vi "FPGA_EncoderOpen & Configure.vi"(4 "IndexActiveHigh":bool=TRUE, 5 "IndexSource":T1={"DevStatus"={"status"=FALSE, "code"=0, "source"=""}, "AnalogTriggerMode?"=FALSE, "DigitalMode"={"DIO Channel"=enum."Disabled"}, "AnalogTriggerMode"={"AnalogTriggerIndex"=enum."Trig 0", "OutputType"=enum."InWindow"}}, 6 "Reverse?":bool, 7 "IndexEdgeSensitive":bool, 8 "error in":errorcluster, 9 "BSource":T1={"DevStatus"={"status"=FALSE, "code"=0, "source"=""}, "AnalogTriggerMode?"=FALSE, "DigitalMode"={"DIO Channel"=enum."Disabled"}, "AnalogTriggerMode"={"AnalogTriggerIndex"=enum."Trig 0", "OutputType"=enum."InWindow"}}, 10 "ASource":T1={"DevStatus"={"status"=FALSE, "code"=0, "source"=""}, "AnalogTriggerMode?"=FALSE, "DigitalMode"={"DIO Channel"=enum."Disabled"}, "AnalogTriggerMode"={"AnalogTriggerIndex"=enum."Trig 0", "OutputType"=enum."InWindow"}}, 11 "EncoderIndex":T5) -> (0 "error out":errorcluster, 3 "Encoder Reference":T6)   [LabVIEW 2017]
uses:
  <vilib>/Rock Robotics/SystemInterfaces/Encoder/FPGA_EncoderDevRef.ctl
  <vilib>/Rock Robotics/SystemInterfaces/Encoder/FPGA_EncoderIdx.ctl
  <vilib>/Rock Robotics/SystemInterfaces/CounterEncoderSourceConvertion/FPGA_CounterEncoderSourceConvertionLVSourceType.ctl
  <vilib>/Rock Robotics/SystemInterfaces/DIO/FPGA_DIODigitalSourceChannel.ctl
  <vilib>/Rock Robotics/SystemInterfaces/AnalogTrigger/FPGA_AnalogTriggerIndex.ctl
  <vilib>/Rock Robotics/SystemInterfaces/AnalogTrigger/FPGA_AnalogTriggerOutType.ctl
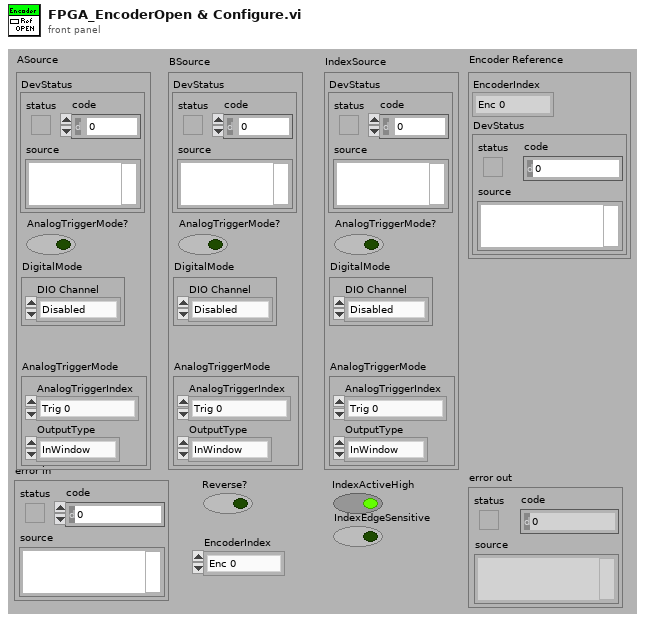
[diagram p1: front panel]
types:
  T1 = typedef "FPGA_CounterEncoderSourceConvertionLVSourceType.ctl" = cluster{"DevStatus":errorcluster, "AnalogTriggerMode?":bool, "DigitalMode":cluster{"DIO Channel":T2}, "AnalogTriggerMode":cluster{"AnalogTriggerIndex":T3, "OutputType":T4}}
  T2 = typedef "FPGA_DIODigitalSourceChannel.ctl" = enum8{"DIO 0", "DIO 1", "DIO 2", "DIO 3", "DIO 4", "DIO 5", "DIO 6", "DIO 7", "DIO 8", "DIO 9", "DIO MXP 0", "DIO MXP 1", "DIO MXP 2", "DIO MXP 3", "DIO MXP 4", "DIO MXP 5", "DIO MXP 6", "DIO MXP 7", "DIO MXP 8", "DIO MXP 9", "DIO MXP 10", "DIO MXP 11", "DIO MXP 12", "DIO MXP 13", "DIO MXP 14", "DIO MXP 15", "Disabled"}
  T3 = typedef "FPGA_AnalogTriggerIndex.ctl" = enum8{"Trig 0", "Trig 1", "Trig 2", "Trig 3", "Trig 4", "Trig 5", "Trig 6", "Trig 7", "Invalid"}
  T4 = typedef "FPGA_AnalogTriggerOutType.ctl" = enum16{"InWindow", "TriggerState", "Rising", "Falling"}
  T5 = typedef "FPGA_EncoderIdx.ctl" = enum8{"Enc 0", "Enc 1", "Enc 2", "Enc 3", "Enc 4", "Enc 5", "Enc 6", "Enc 7", "Invalid"}
  T6 = typedef "FPGA_EncoderDevRef.ctl" = cluster{"EncoderIndex":T5, "DevStatus":errorcluster}
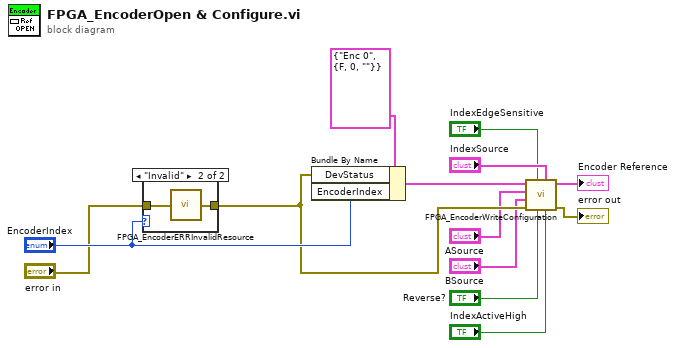
[diagram p0: block diagram]
diagram:
  n1 = case shown="\"Invalid\"" "EncoderIndex" {
    tunnel: [w14 w16] -> w9
    tunnel: "error in" -> [w14 w15]
    frame Default {
    }
    frame "Invalid" {
      n2 = call <vilib>:"FPGA_EncoderERRInvalidResource.vi"("error in (no error)"=w15) -> ("error out"=w16:errorcluster)
    }
  }
  n3 = Bundle By Name(cluster=T6 {"EncoderIndex"=enum."Enc 0", "DevStatus"={"status"=FALSE, "code"=0, "source"=""}} ("Encoder Reference out"), "DevStatus"=w9, "EncoderIndex"="EncoderIndex") -> (w11:T6)
  n4 = call <vilib>:"FPGA_EncoderWriteConfiguration.vi"("IndexActiveHigh"="IndexActiveHigh", "IndexSource"="IndexSource", "Reverse?"="Reverse?", "IndexEdgeSensitive"="IndexEdgeSensitive", "error in (no error)"=w9, "BSource"="BSource", "ASource"="ASource", "EncoderDevRef"=w11) -> ("error out"=→"error out":errorcluster, "EncoderDevRef"=→"Encoder Reference":T6)  [unwired: 2 out]
